vi "PCO_RecorderSetCompressionParams.vi"(0 "phRec":u64, 5 "phCam":u64, 7 "strCompressionParams":T1, 11 "error in (no error)":errorcluster {"code" format="%x"}) -> (4 "phRec out":u64, 6 "ErrorMessage":i32 format="%x", 15 "error out":errorcluster {"code" format="%x"})   [LabVIEW 2019, in "Recorder.lvlib"]
doc: "int WINAPI PCO_RecorderSetCompressionParams(HANDLE phRec, HANDLE phCam, PCO_Recorder_CompressionParams strCompressionParams);"
uses:
  Recorder.lvlib
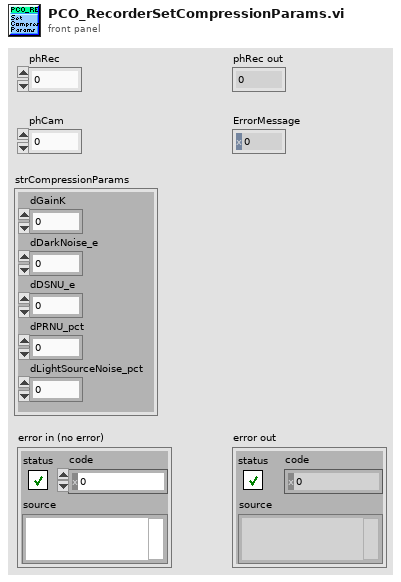
[diagram p1: front panel]
types:
  T1 = cluster{"dGainK":dbl, "dDarkNoise_e":dbl, "dDSNU_e":dbl, "dPRNU_pct":dbl, "dLightSourceNoise_pct":dbl}
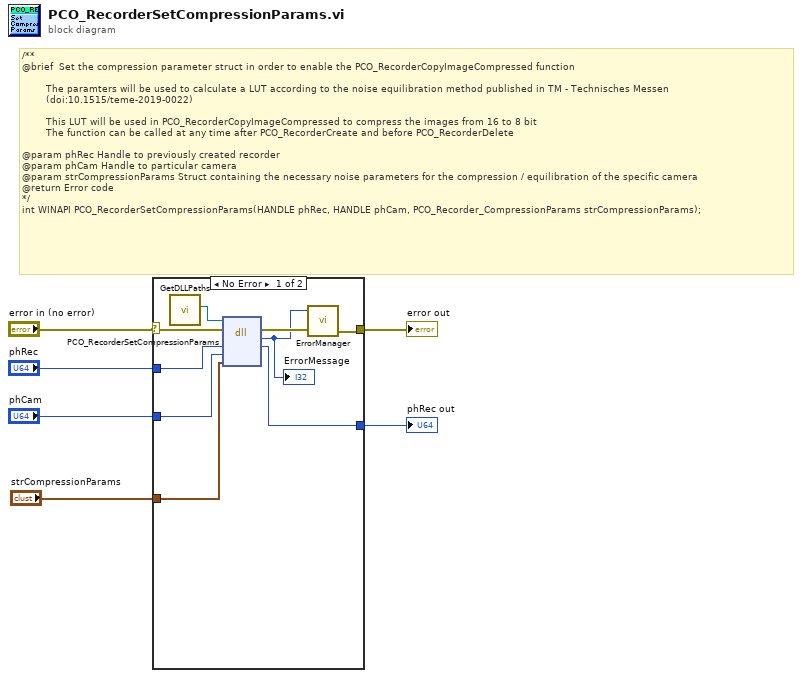
[diagram p0: block diagram]
diagram:
  # "/**\n@brief  Set the compression parameter struct in order to enable the PCO_RecorderCopyImageCompressed function\n\n        The paramters will be used to calculate a LUT according to the noise equilibration method published in TM - Technisches Messen \n        (doi:10.1515/teme-2019-0022)\n\n        This LUT will be used in PCO_RecorderCopyImageCompressed to compress the images from 16 to 8 bit\n        The function can be called at any time after PCO_RecorderCreate and before PCO_RecorderDelete\n\n@param phRec Handle to previously created recorder\n@param phCam Handle to particular camera\n@param strCompressionParams Struct containing the necessary noise parameters for the compression / equilibration of the specific camera\n@return Error code\n*/\nint WINAPI PCO_RecorderSetCompressionParams(HANDLE phRec, HANDLE phCam, PCO_Recorder_CompressionParams strCompressionParams);"
  n1 = case shown="No Error" "error in (no error)" {
    selector: "error in (no error)" -> [w11 w16]
    tunnel: "phRec" -> [w15 w17]
    tunnel: [w14 w17] -> w5
    tunnel: "phCam" -> [w13 _]
    tunnel: [w9 w16] -> w3
    tunnel: "strCompressionParams" -> [w7 _]
    frame No Error {
      n2 = call "GetDLLPaths.vi"() -> ("PCO_Recorder_Path"=w12:path)  [unwired: 9 in, 2 out]
      n3 = dll-call lib="?" fn="PCO_RecorderSetCompressionParams"(path in=w12, error in=w11, "phRec"=w15, "phCam"=w13, "strCompressionParams"=w7) -> (error out=w10:errorcluster, "return type"=w8:i32, "phRec"=w14:u64)  [unwired: 3 in, 1 out]
      "ErrorMessage" <- w8
      n4 = call "ErrorManager.vi"("error in (no error)"=w10, "error code"=w8) -> ("error out"=w9:errorcluster)  [unwired: 3 in]
    }
    frame Error {
    }
  }
  "phRec out" <- w5
  "error out" <- w3
